vi "Header.vi"(0 "Sample":string, 1 "User":string, 3 "File Path":path) -> (2 "File Path":path)   [LabVIEW 2013]
uses:
  <vilib>/Utility/file.llb/Write To Spreadsheet File (string).vi
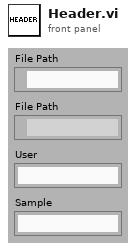
[diagram p1: front panel]
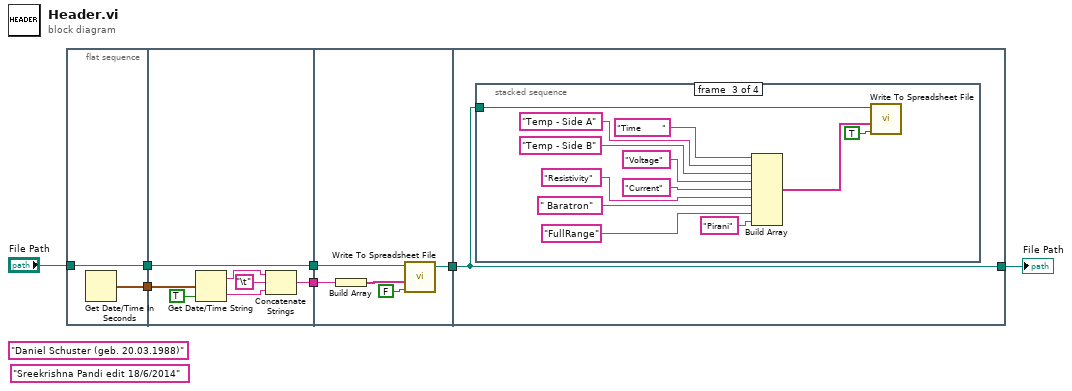
[diagram p0: block diagram]
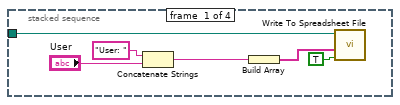
[diagram p2: hidden frame]
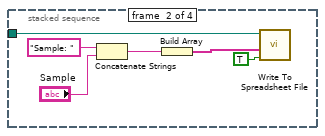
[diagram p3: hidden frame]
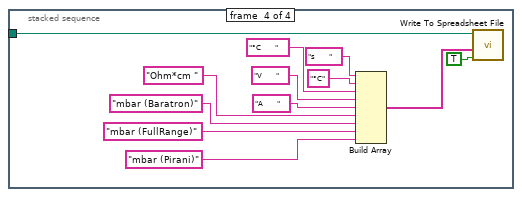
[diagram p4: hidden frame]
diagram:
  (unwired) "Sreekrishna Pandi edit 18/6/2014"
  (unwired) "Daniel Schuster (geb. 20.03.1988)"
  n1 = flat-sequence {
    tunnel: [w8] -> w7
    tunnel: [w9] -> w6
    tunnel: "File Path" -> [w9]
    tunnel: w7 -> [w14]
    tunnel: [w13] -> w5
    tunnel: [w10] -> w4
    tunnel: w6 -> [w10]
    tunnel: w5 -> [w20]
    tunnel: w4 -> [w18]
    tunnel: [w17] -> w1
    tunnel: [w22] -> w2
    tunnel: w1 -> [w22]
    frame #0 {
      n2 = Get Date/Time In Seconds() -> (seconds since 1Jan1904=w8:timestamp)
    }
    frame #1 {
      n3 = Get Date/Time String(seconds (now)=w14, want seconds? (F)=TRUE) -> (date string=w16:string, time string=w12:string)  [unwired: 1 in]
      n4 = Concatenate Strings(w16, "\t", w12) -> (w13:string)
    }
    frame #2 {
      n5 = Build Array(w20) -> (w19:string[])
      n6 = call-poly <vilib>:"Write To Spreadsheet File.vi"("append to file? (new file:F)"=FALSE ("transpose? (no:F)"), "1D data"=w19, "file path (dialog if empty)"=w18) -> ("new file path (Not A Path if cancelled)"=w17:path)  [unwired: 5 in]
    }
    frame #3 {
      n7 = stacked-sequence {
        tunnel: w22 -> [w26 w32 w35 w51]
        frame #0 {
          n8 = Concatenate Strings("User: ", "User") -> (w25:string)
          n9 = Build Array(w25) -> (w27:string[])
          n10 = call-poly <vilib>:"Write To Spreadsheet File.vi"("append to file? (new file:F)"=TRUE ("transpose? (no:F)"), "1D data"=w27, "file path (dialog if empty)"=w26) -> ()  [unwired: 5 in, 1 out]
        }
        frame #1 {
          n11 = Concatenate Strings("Sample: ", "Sample") -> (w31:string)
          n12 = Build Array(w31) -> (w33:string[])
          n13 = call-poly <vilib>:"Write To Spreadsheet File.vi"("append to file? (new file:F)"=TRUE ("transpose? (no:F)"), "1D data"=w33, "file path (dialog if empty)"=w32) -> ()  [unwired: 5 in, 1 out]
        }
        frame #2 {
          n14 = Build Array("Time       ", "Temp - Side A", "Temp - Side B" ("element"), "Voltage", "Current", "Resistivity", " Baratron", "FullRange", "Pirani") -> (w39:string[])
          n15 = call-poly <vilib>:"Write To Spreadsheet File.vi"("append to file? (new file:F)"=TRUE ("transpose? (no:F)"), "1D data"=w39, "file path (dialog if empty)"=w35) -> ()  [unwired: 5 in, 1 out]
        }
        frame #3 {
          n16 = Build Array("s       ", "°C" ("element"), "°C       ", "V       ", "A       ", "Ohm*cm ", "mbar (Baratron)", "mbar (FullRange)", "mbar (Pirani)") -> (w52:string[])
          n17 = call-poly <vilib>:"Write To Spreadsheet File.vi"("append to file? (new file:F)"=TRUE ("transpose? (no:F)"), "1D data"=w52, "file path (dialog if empty)"=w51) -> ()  [unwired: 5 in, 1 out]
        }
      }
    }
  }
  "File Path" <- w2
